vi "2 station_keeping_circles.vi"(10 "Mission in":refnum<class "Mission.lvclass">) -> (2 "No Sail Circles":T1[](array[typedef]))   [LabVIEW 2011]
uses:
  2 Classes/Mission/Mission.lvclass
  2 Typedefs/UTM Circle.ctl
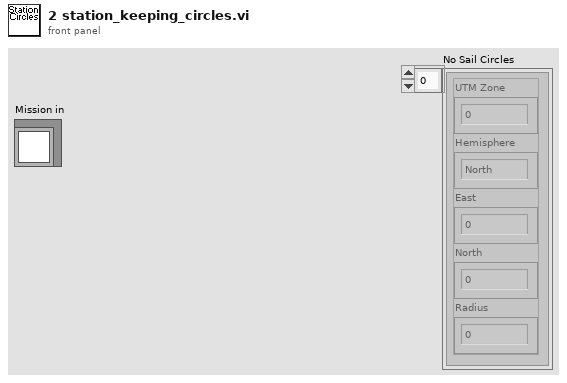
[diagram p1: front panel]
types:
  T1 = typedef "UTM Circle.ctl" = cluster{"UTM Zone":dbl, "Hemisphere":enum16{"North", "South"}, "East":dbl, "North":dbl, "Radius":dbl}
  T2 = typedef "UTM Location.ctl" = cluster{"UTM Zone":dbl, "Hemisphere":enum16{"North", "South"}, "East":dbl, "North":dbl}
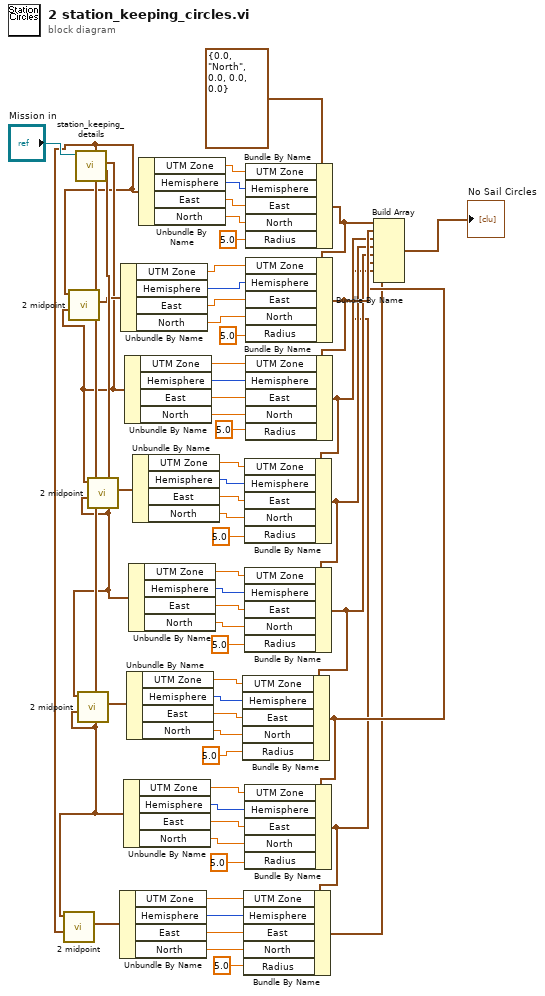
[diagram p0: block diagram]
diagram:
  n1 = call-dynamic "station_keeping_details.vi"("Mission in"="Mission in") -> ("Buoy SE"=w4:T2, "Buoy NE"=w2:T2, "Buoy SW"=w6:T2, "Buoy NW"=w1:T2)  [unwired: 4 in, 3 out]
  n2 = call "2 midpoint.vi"("UTM 2"=w1, "UTM 1"=w6) -> ("Midpoint"=w8:T2)  [unwired: 9 in]
  n3 = call "2 midpoint.vi"("UTM 2"=w2, "UTM 1"=w1) -> ("Midpoint"=w3:T2)  [unwired: 9 in]
  n4 = call "2 midpoint.vi"("UTM 2"=w6, "UTM 1"=w4) -> ("Midpoint"=w7:T2)  [unwired: 9 in]
  n5 = call "2 midpoint.vi"("UTM 2"=w4, "UTM 1"=w2) -> ("Midpoint"=w5:T2)  [unwired: 9 in]
  n6 = Unbundle By Name(w8) -> ("UTM Zone"=w29:dbl, "Hemisphere"=w30:enum16{"North", "South"}, "East"=w31:dbl, "North"=w32:dbl)
  n7 = Unbundle By Name(w3) -> ("UTM Zone"=w36:dbl, "Hemisphere"=w35:enum16{"North", "South"}, "East"=w34:dbl, "North"=w33:dbl)
  n8 = Unbundle By Name(w6) -> ("UTM Zone"=w25:dbl, "Hemisphere"=w26:enum16{"North", "South"}, "East"=w27:dbl, "North"=w28:dbl)
  n9 = Unbundle By Name(w2) -> ("UTM Zone"=w9:dbl, "Hemisphere"=w10:enum16{"North", "South"}, "East"=w11:dbl, "North"=w12:dbl)
  n10 = Unbundle By Name(w7) -> ("UTM Zone"=w21:dbl, "Hemisphere"=w22:enum16{"North", "South"}, "East"=w23:dbl, "North"=w24:dbl)
  n11 = Unbundle By Name(w4) -> ("UTM Zone"=w17:dbl, "Hemisphere"=w18:enum16{"North", "South"}, "East"=w19:dbl, "North"=w20:dbl)
  n12 = Unbundle By Name(w5) -> ("UTM Zone"=w13:dbl, "Hemisphere"=w14:enum16{"North", "South"}, "East"=w15:dbl, "North"=w16:dbl)
  n13 = Unbundle By Name(w1) -> ("UTM Zone"=w56:dbl, "Hemisphere"=w55:enum16{"North", "South"}, "East"=w54:dbl, "North"=w53:dbl)
  n14 = Bundle By Name(cluster=T1 {"UTM Zone"=0.0, "Hemisphere"=enum."North", "East"=0.0, "North"=0.0, "Radius"=0.0} ("UTM Location"), "UTM Zone"=w56, "Hemisphere"=w55, "East"=w54, "North"=w53, "Radius"=5.0) -> (w51:T1)
  n15 = Bundle By Name(cluster=w51, "UTM Zone"=w36, "Hemisphere"=w35, "East"=w34, "North"=w33, "Radius"=5.0) -> (w50:T1)
  n16 = Bundle By Name(cluster=w50, "UTM Zone"=w9, "Hemisphere"=w10, "East"=w11, "North"=w12, "Radius"=5.0) -> (w49:T1)
  n17 = Bundle By Name(cluster=w49, "UTM Zone"=w13, "Hemisphere"=w14, "East"=w15, "North"=w16, "Radius"=5.0) -> (w48:T1)
  n18 = Bundle By Name(cluster=w48, "UTM Zone"=w17, "Hemisphere"=w18, "East"=w19, "North"=w20, "Radius"=5.0) -> (w47:T1)
  n19 = Bundle By Name(cluster=w47, "UTM Zone"=w21, "Hemisphere"=w22, "East"=w23, "North"=w24, "Radius"=5.0) -> (w46:T1)
  n20 = Bundle By Name(cluster=w46, "UTM Zone"=w25, "Hemisphere"=w26, "East"=w27, "North"=w28, "Radius"=5.0) -> (w44:T1)
  n21 = Bundle By Name(cluster=w44, "UTM Zone"=w29, "Hemisphere"=w30, "East"=w31, "North"=w32, "Radius"=5.0) -> (w45:T1)
  n22 = Build Array(w51, w50, w49, w48, w47, w46, w44, w45) -> (→"No Sail Circles":T1[])
